vi "BWC_CollectBeamImagingCalibration.vi"() -> ()   [LabVIEW 2017]
panel:
  in  "Command To Write 4":string="NORM"
  out "error out 5":errorcluster={"status"=FALSE, "code"=0, "source"="Response\nindicates valid\n command."}
  out "Completion Response  6":string=">"
  out "Acknowledge Response 6":string="@"
  in  "Command To Write 3":string="SRON 0"
  out "concatenated string 3":string="C:\\Users\\1TEM\\Documents\\1TEM_control\\tem_image_acquisition\\bin\\Release\\tem_image_acquisition.exe --gain 50 --exposure 1000 --blacklvl 180 --filename \"calib_SPOT_1024__768_capture.png\""
  out "standard error":string
  out "concatenated string 2":string="--gain 50 --exposure 1000 --blacklvl 180 --filename \"calib_SPOT_1024__768_capture.png\""
  out "standard output":string="Initializing camera ...\r\nSuccess!\r\nGetting sensor info ...\r\nSuccess!\r\nCamera ID: 1\r\nSensor dimensions: 1600 x 1200 (assuming bit-depth per pixel of 24)\r\nAllocating memory for images ...\r\nSuccess!\r\nSetting image memory location ...\r\nSuccess!\r\nGetting current exposure ...\r\nSuccess!\r\nCurrent exposure: 25.1076 ms\r\nGetting current frame rate ...\r\nSuccess!\r\nCurrent frame rate 39.7962\r\n\r\nSuccess!\r\nSuccess!\r\nSuccess!\r\nSetting frame rate to 0.1 fps ...\r\nSuccess!\r\nFrame rate set to 0.99985 fps ...\r\n\r\nGetting valid exposure range ...\r\nSuccess!\r\nMin: 0.0201 ms\r\nMax: 999.98 ms\r\nInc: 0.170122 ms\r\nSetting new exposure to: 1000 ms ...\r\nSuccess!\r\nCurrent exposure now 999.98 ms\r\n\r\nGetting current gain ...\r\nCurrent gain setting is: 0\r\nSuccess!\r\nSetting gain to 50 ...\r\nSuccess!\r\nGetting current gain ...\r\nCurrent gain setting is: 50\r\n\r\nSuccess!\r\nGetting current blacklevel ...\r\nSuccess!\r\nCurrent blacklevel: 132\r\nSetting blacklevel to 180...\r\nSuccess!\r\nGetting current blacklevel ...\r\nSuccess!\r\nCurrent blacklevel: 180\r\n\r\nFreezing video ...\r\nSuccess!\r\n\r\nFreezing video ...\r\nSuccess!\r\n\r\nSaving image ...\r\n\r\nSaving image to calib_SPOT_1024__768_capture.png ...\r\nSuccess!\r\n\r\nShutting down camera ...\r\n"
  in  "ImagePath":path=path "\\\\LEO1272\\Caplins/Calibrations"
  in  "opts":string="--gain 50 --exposure 1000 --blacklvl 180"
  in  "program name":string="tem_image_acquisition.exe"
  in  "program path":path=path "C:/Users/1TEM/Documents/1TEM_control/tem_image_acquisition/bin/Release"
  out "concatenated string":string="SPOT 1024  768"
  out "error out 4":errorcluster={"status"=FALSE, "code"=0, "source"="Response\nindicates valid\n command."}
  out "Completion Response  5":string=">"
  out "Acknowledge Response 5":string="@"
  in  "Y pix step":i32=256
  in  "X pix step":i32=256
  out "Pixel Size":dbl=2826.855455 format="%#_12g"
  out "error out 3":errorcluster={"status"=FALSE, "code"=0, "source"="Response\nindicates valid\n command."}
  out "Completion Response  4":string=">2826.855455"
  out "Acknowledge Response 4":string="@"
  in  "Command To Write 2":string="PIX?"
  out "error out 2":errorcluster={"status"=FALSE, "code"=0, "source"="Response\nindicates valid\n command."}
  out "Completion Response  3":string=">"
  out "Acknowledge Response 3":string="@"
  in  "Command To Write":string="MAG 100"
  out "Completion Response  2":string=">"
  out "Acknowledge Response 2":string="@"
  out "error out":errorcluster={"status"=FALSE, "code"=0, "source"="Response\nindicates valid\n command."}
  in  "VISA resource name":refnum<visa-resource-name>="COM4"
  # "Steps:\n1. Request and Set MAG\n2. Get pixel size (Make sure 1024x768 images)\n3. For a grid of points:\n        Spot Mode\n        Collect Image\n        Save Image\n4. Ideally, do analysis... but maybe matlab/octave is easier..."
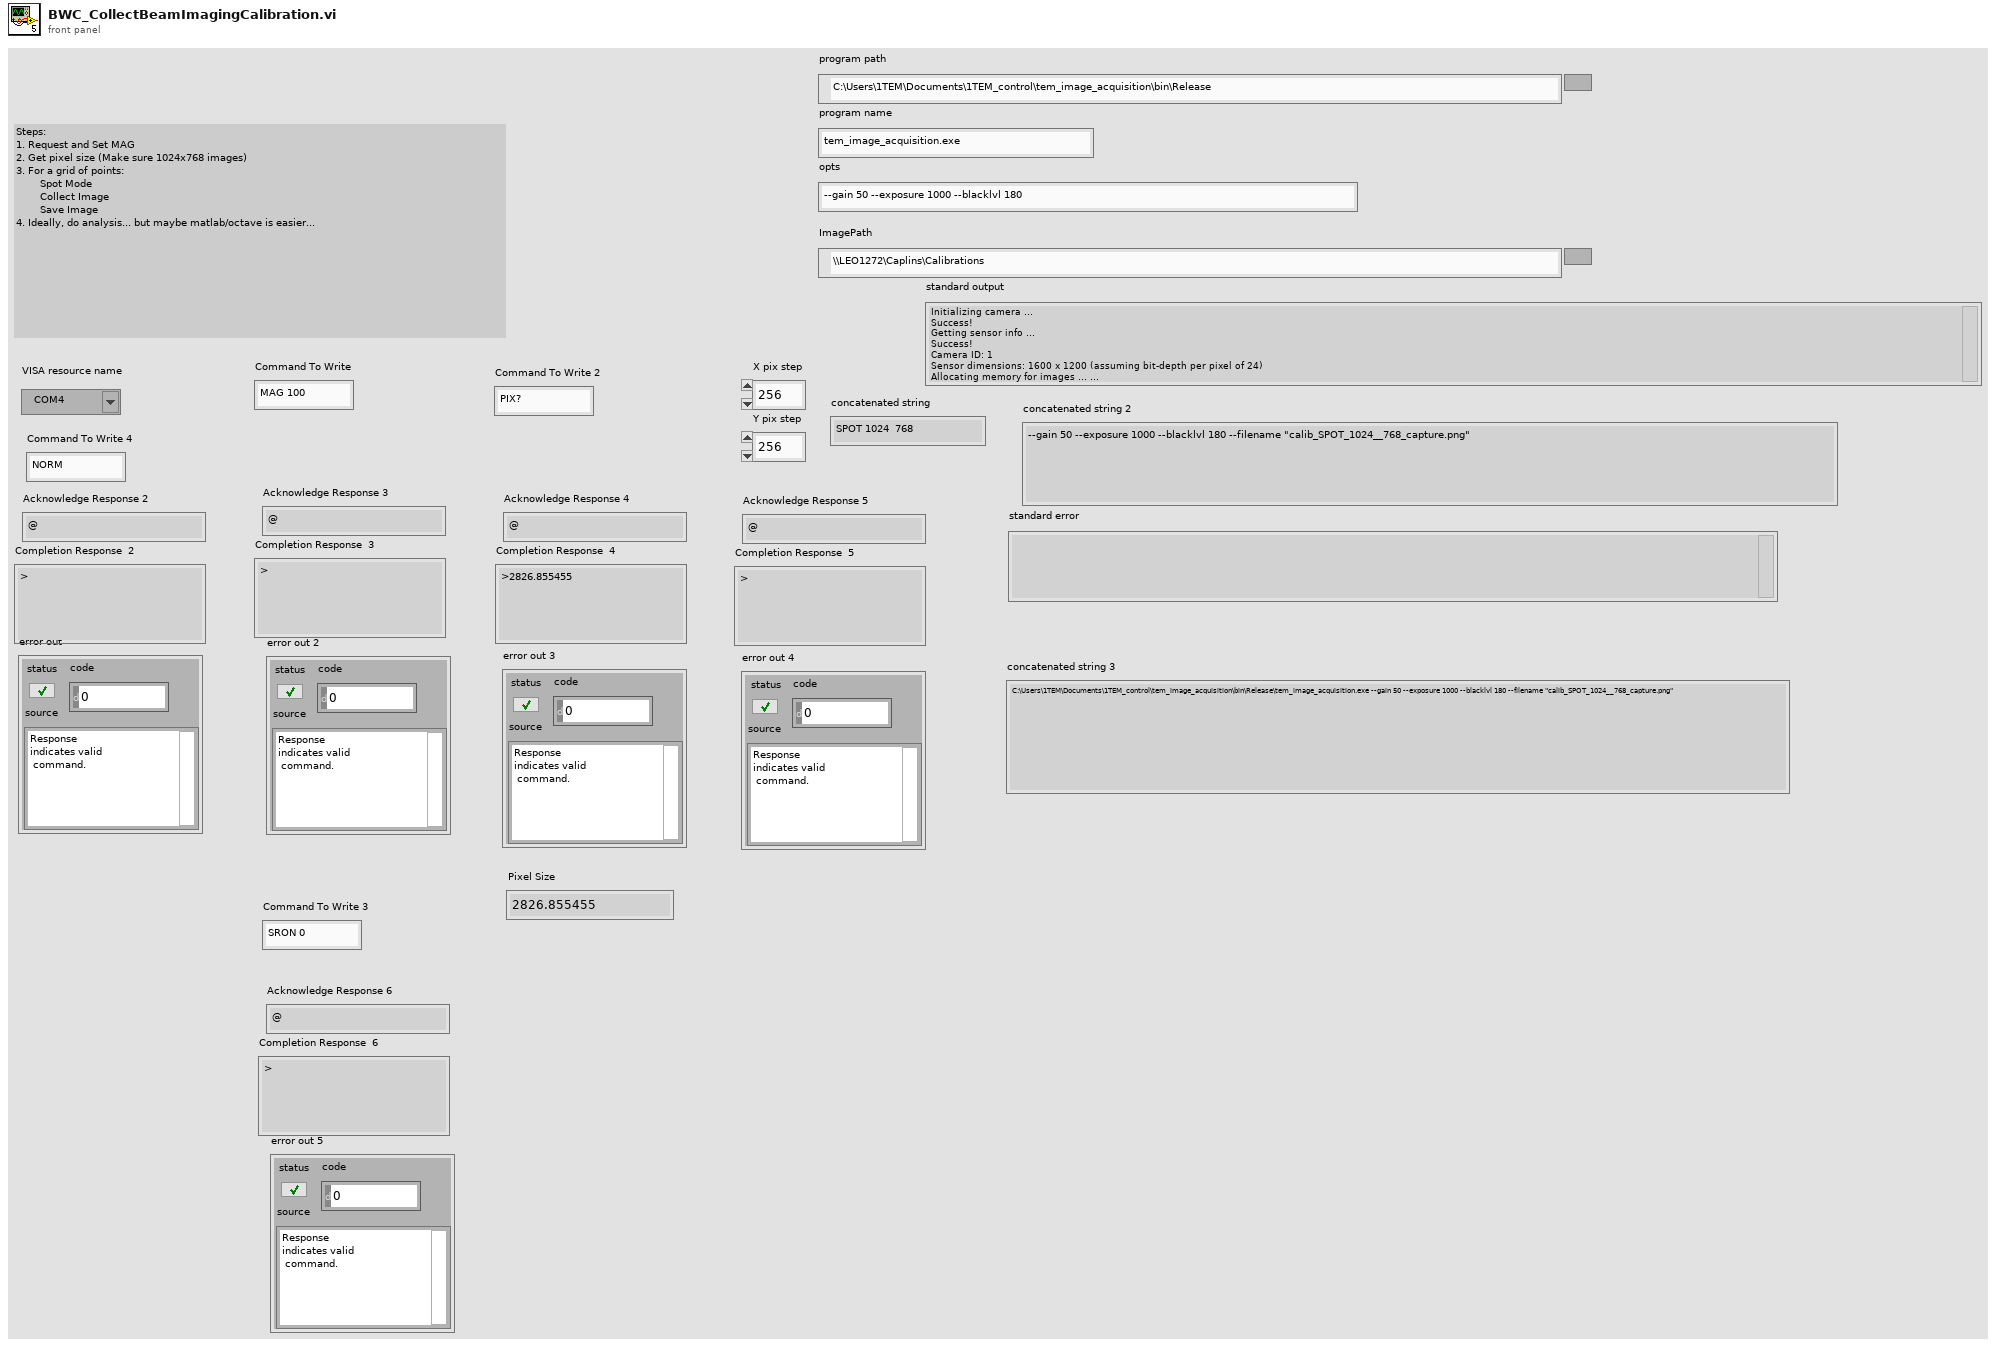
[diagram p1: front panel]
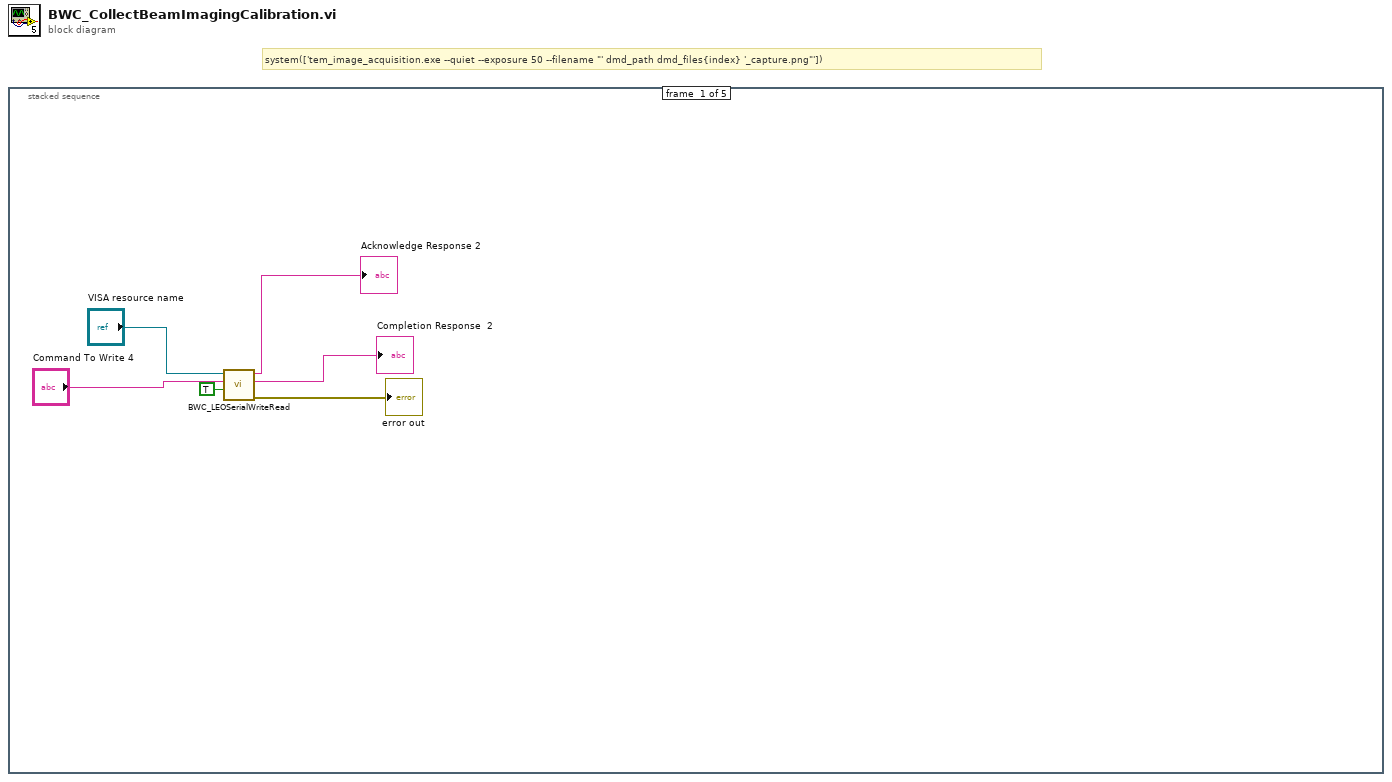
[diagram p0: block diagram]
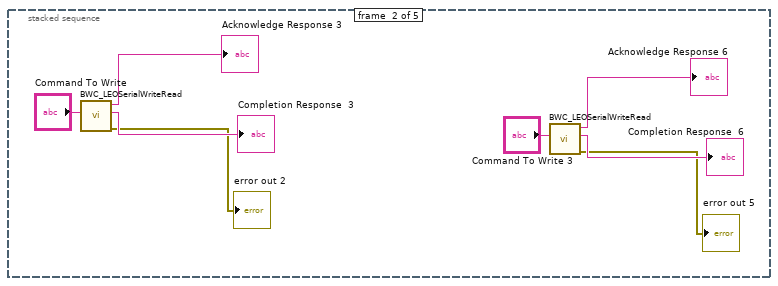
[diagram p2: hidden frame]
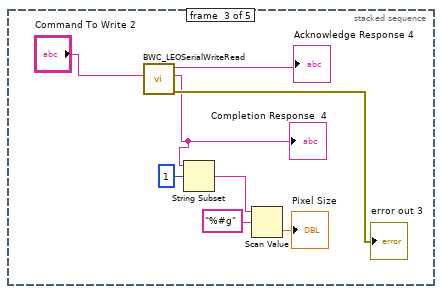
[diagram p3: hidden frame]
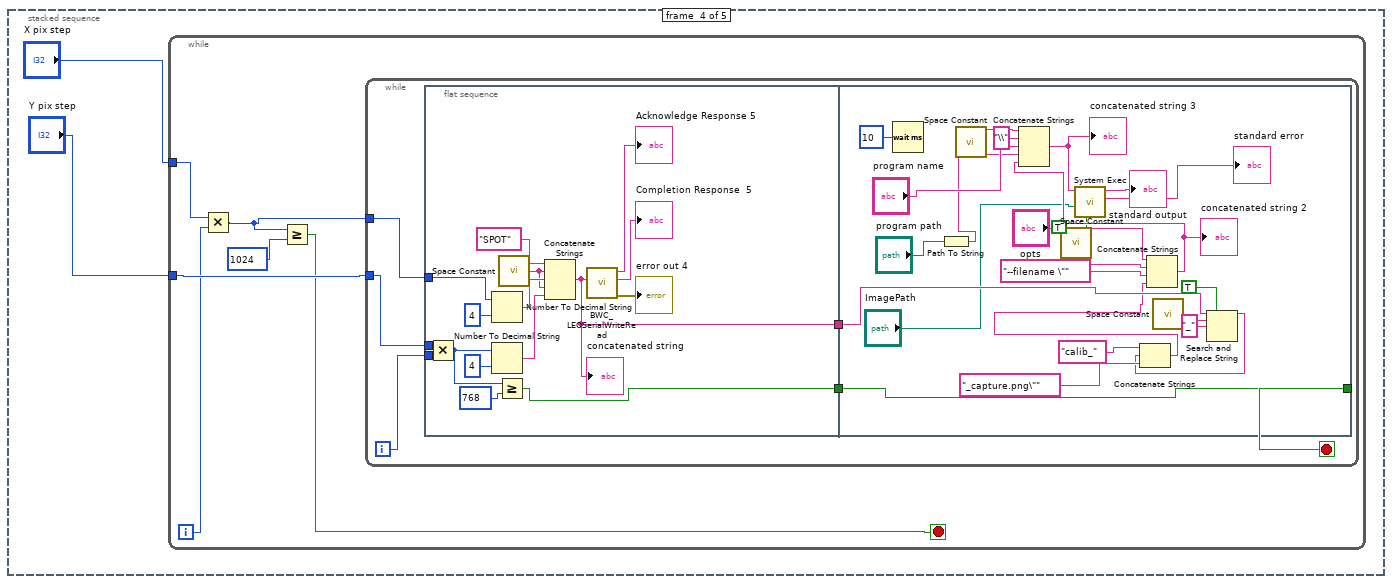
[diagram p4: hidden frame]
diagram:
  # "system(['tem_image_acquisition.exe --quiet --exposure 50 --filename \"' dmd_path dmd_files{index} '_capture.png\"'])"
  n1 = stacked-sequence {
    frame #0 {
      n2 = call "BWC_LEOSerialWriteRead.vi"("Perform Two Reads Following Write"=TRUE, "Command To Write"="Command To Write 4", "VISA resource name"="VISA resource name") -> ("error out"=→"error out":errorcluster, "Completion Response"=→"Completion Response  2":string, "Acknowledge Response"=→"Acknowledge Response 2":string)  [unwired: 4 in, 1 out]
    }
    frame #1 {
      n3 = call "BWC_LEOSerialWriteRead.vi"("Command To Write"="Command To Write") -> ("error out"=→"error out 2":errorcluster, "Completion Response"=→"Completion Response  3":string, "Acknowledge Response"=→"Acknowledge Response 3":string)  [unwired: 6 in, 1 out]
      n4 = call "BWC_LEOSerialWriteRead.vi"("Command To Write"="Command To Write 3") -> ("error out"=→"error out 5":errorcluster, "Completion Response"=→"Completion Response  6":string, "Acknowledge Response"=→"Acknowledge Response 6":string)  [unwired: 6 in, 1 out]
    }
    frame #2 {
      n5 = call "BWC_LEOSerialWriteRead.vi"("Command To Write"="Command To Write 2") -> ("error out"=→"error out 3":errorcluster, "Completion Response"=w19:string, "Acknowledge Response"=→"Acknowledge Response 4":string)  [unwired: 6 in, 1 out]
      "Completion Response  4" <- w19
      n6 = String Subset(string=w19, offset (0)=1) -> (substring=w17:string)  [unwired: 1 in]
      n7 = Scan Value(string=w17, format string="%#g") -> (value=→"Pixel Size":dbl)  [unwired: 1 in, 1 out]
    }
    frame #3 {
      n8 = while {
        tunnel: "Y pix step" -> [w30]
        tunnel: "X pix step" -> [w29]
        i -> [w28]
        stop <- w26 stop-if-true
        n9 = Multiply(x=w29, y=w28) -> (x*y=w25:i32)
        n10 = Greater Or Equal?(x=w25, y=1024) -> (x >= y?=w26:bool)
        n11 = while {
          tunnel: w25 -> [w33]
          tunnel: w30 -> [w36]
          i -> [w35]
          stop <- w34 stop-if-true
          n12 = flat-sequence {
            tunnel: w36 -> [w52]
            tunnel: w35 -> [w51]
            tunnel: [w49] -> w32
            tunnel: w33 -> [w46]
            tunnel: [w37] -> w31
            tunnel: [w74] -> w34
            tunnel: w32 -> [w74]
            tunnel: w31 -> [w67]
            frame #0 {
              n13 = Multiply(x=w52, y=w51) -> (x*y=w45:i32)
              n14 = Number To Decimal String(number=w46, width (-)=i16 4) -> (decimal integer string=w44:string)
              n15 = Number To Decimal String(number=w45, width (-)=i16 4) -> (decimal integer string=w42:string)
              n16 = Greater Or Equal?(x=w45, y=768) -> (x >= y?=w49:bool)
              n17 = call <vilib>:"Space Constant.vi"() -> ("String"=w41:string)
              n18 = Concatenate Strings("SPOT" ("Command To Write"), w41, w44, w41, w42) -> (w37:string)
              "concatenated string" <- w37
              n19 = call "BWC_LEOSerialWriteRead.vi"("Command To Write"=w37) -> ("error out"=→"error out 4":errorcluster, "Completion Response"=→"Completion Response  5":string, "Acknowledge Response"=→"Acknowledge Response 5":string)  [unwired: 6 in, 1 out]
            }
            frame #1 {
              n20 = Wait (ms)(milliseconds to wait=u32 10) -> ()  [unwired: 1 out]
              n21 = Path To String(path="program path") -> (string=w55:string)
              n22 = call <vilib>:"Space Constant.vi"() -> ("String"=w60:string)
              n23 = call <vilib>:"Space Constant.vi"() -> ("String"=w69:string)
              n24 = call <vilib>:"Space Constant.vi"() -> ("String"=w65:string)
              n25 = Search and Replace String(replace all?=TRUE ("replace all? (F)"), input string=w67, search string=w65, replace string="_" ("replace string (\"\")")) -> (result string=w63:string)  [unwired: 4 in, 3 out]
              n26 = Concatenate Strings("calib_", w63, "_capture.png\"" ("string")) -> (w57:string)
              n27 = Concatenate Strings("opts", w69, "--filename \"", w57) -> (w61:string)
              "concatenated string 2" <- w61
              n28 = Concatenate Strings(w55, "\\" ("string"), "program name", w60, w61) -> (w59:string)
              "concatenated string 3" <- w59
              n29 = call <vilib>:"System Exec.vi"("run minimized? (F)"=TRUE, "working directory"="ImagePath", "command line"=w59) -> ("standard error"=→"standard error":string, "standard output"=→"standard output":string)  [unwired: 5 in, 2 out]
            }
          }
        }
      }
    }
    frame #4 {
    }
  }
